vi "Multiclamp Auto Tune Gain.vi"(6 "Target Delta pp":dbl, 8 "error in (no error)":errorcluster, 9 "pnError":i32, 10 "Multiclamp Reference":i32, 11 "Test Signal":waveform(dbl)) -> (0 "error out":errorcluster, 1 "pnError out":i32, 2 "Multiclamp Reference Out":i32, 3 "Test Signal Out":waveform(dbl))   [LabVIEW 2012, in "MultiClamp 700B Controls.lvlib"]
uses:
  MultiClamp 700B Controls.lvlib
  <vilib>/measure/mascope.llb/Amplitude and Levels 1 chan.vi
  AxMultiClampMsg/AxMultiClampMsg.lvlib
  <vilib>/measure/NI_MAPro.lvlib
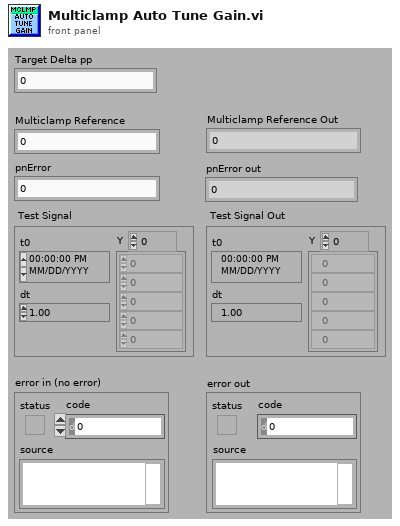
[diagram p1: front panel]
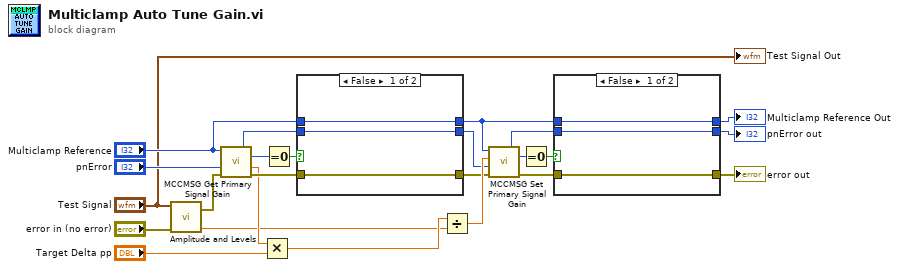
[diagram p0: block diagram]
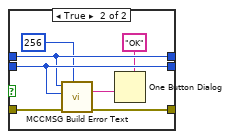
[diagram p2: hidden frame]
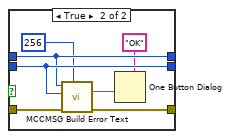
[diagram p3: hidden frame]
diagram:
  n1 = call-poly <vilib>:"Amplitude and Levels.vi"("error in (no error)"="error in (no error)", "signal in"="Test Signal") -> ("error out"=w2:errorcluster, "amplitude"=w4:dbl)  [unwired: 6 in, 2 out]
  n2 = call "MCCMSG Get Primary Signal Gain.vi"("error in (no error)"=w2, "pnError"="pnError", "hMCCmsg"="Multiclamp Reference") -> ("error out"=w20:errorcluster, "pnError out"=w18:i32, "pdGain out"=w6:dbl, "function return"=w19:i32)  [unwired: 5 in]
  n3 = Multiply(x=w6, y="Target Delta pp") -> (x*y=w24:dbl)
  n4 = Equal To 0?(x=w19) -> (x = 0?=w21:bool)
  n5 = case shown="False" w21 {
    tunnel: w18 -> [w27 w33]
    tunnel: w20 -> [w25 w34]
    tunnel: "Multiclamp Reference" -> [w26 w32]
    tunnel: [w27 w33] -> w14
    tunnel: [w26 w32] -> w10
    tunnel: [w25 w28] -> w15
    frame False {
    }
    frame True {
      n6 = call "MCCMSG Build Error Text.vi"("uMaxLen"=u32 256, "error in (no error)"=w34, "nErrorNum"=w33, "hMCCmsg"=w32) -> ("error out"=w28:errorcluster, "sTxtBuf out"=w31:string)  [unwired: 5 in, 1 out]
      n7 = One Button Dialog(message=w31, button name ("OK")="OK") -> ()  [unwired: 1 out]
    }
  }
  n8 = Divide(x=w24, y=w4) -> (x/y=w23:dbl)
  n9 = call "MCCMSG Set Primary Signal Gain.vi"("error in (no error)"=w15, "pnError"=w14, "dGain"=w23, "hMCCmsg"=w10) -> ("error out"=w13:errorcluster, "pnError out"=w11:i32, "function return"=w12:i32)  [unwired: 5 in]
  n10 = Equal To 0?(x=w12) -> (x = 0?=w22:bool)
  n11 = case shown="False" w22 {
    tunnel: w11 -> [w37 w43]
    tunnel: w13 -> [w35 w44]
    tunnel: w10 -> [w36 w42]
    tunnel: [w37 w43] -> w8
    tunnel: [w36 w42] -> w7
    tunnel: [w35 w38] -> w9
    frame False {
    }
    frame True {
      n12 = call "MCCMSG Build Error Text.vi"("uMaxLen"=u32 256, "error in (no error)"=w44, "nErrorNum"=w43, "hMCCmsg"=w42) -> ("error out"=w38:errorcluster, "sTxtBuf out"=w41:string)  [unwired: 5 in, 1 out]
      n13 = One Button Dialog(message=w41, button name ("OK")="OK") -> ()  [unwired: 1 out]
    }
  }
  "Multiclamp Reference Out" <- w7
  "pnError out" <- w8
  "error out" <- w9
  "Test Signal Out" <- "Test Signal"
